vi "RSA Generate Keys.vi"(8 "error in (no error)":errorcluster, 11 "RSA in":refnum<class "RSA.lvclass">) -> (0 "error out":errorcluster, 1 "public_key":string, 2 "private_key":string, 3 "RSA out":refnum<class "RSA.lvclass">)   [LabVIEW 2021, in "RSA.lvclass"]
uses:
  RSA.lvclass
  RSA.lvclass/RSA.ctl
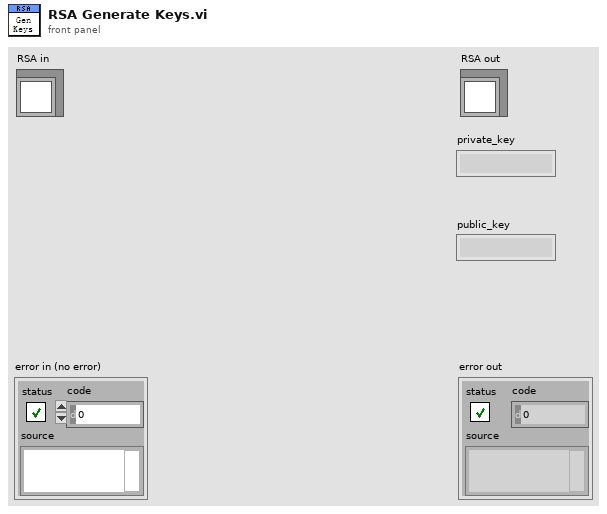
[diagram p1: front panel]
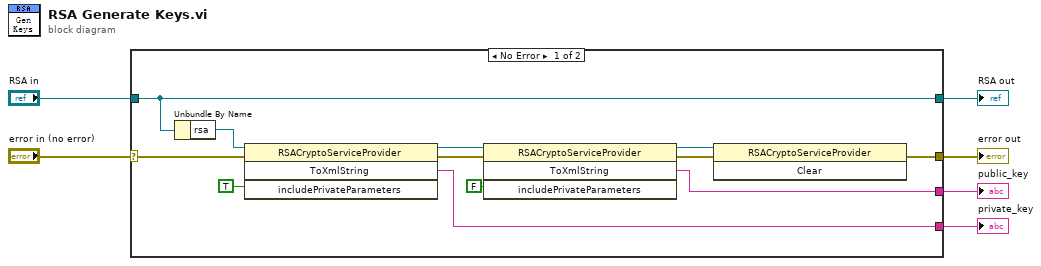
[diagram p0: block diagram]
diagram:
  n1 = case shown="No Error" "error in (no error)" {
    selector: "error in (no error)" -> [w7 w20]
    tunnel: [w12 w20] -> w5
    tunnel: [w9 w19] -> w3
    tunnel: "RSA in" -> [w9 w19]
    tunnel: [w11 _] -> w2
    tunnel: [w10 _] -> w1
    frame No Error {
      n2 = Unbundle By Name(w9) -> ("rsa"=w8:refnum<k24>)
      n3 = invoke class="RSACryptoServiceProvider" method="ToXmlString"(reference=w8, error in=w7, "includePrivateParameters"=TRUE) -> (reference out=w15:refnum<k24>, error out=w16:errorcluster, "ToXmlString"=w10:string)  [unwired: 1 in, 1 out]
      n4 = invoke class="RSACryptoServiceProvider" method="ToXmlString"(reference=w15, error in=w16, "includePrivateParameters"=FALSE) -> (reference out=w17:refnum<k24>, error out=w18:errorcluster, "ToXmlString"=w11:string)  [unwired: 1 in, 1 out]
      n5 = invoke class="RSACryptoServiceProvider" method="Clear"(reference=w17, error in=w18) -> (error out=w12:errorcluster)  [unwired: 1 in, 2 out]
    }
    frame Error {
    }
  }
  "error out" <- w5
  "RSA out" <- w3
  "public_key" <- w2
  "private_key" <- w1
